vi "报警信息.vi"(8 "error in (no error)":errorcluster, 11 "data":T1) -> (0 "error out":errorcluster)   [LabVIEW 2016, in "MB SLAVE.lvlib"]
uses:
  MB SLAVE.lvlib
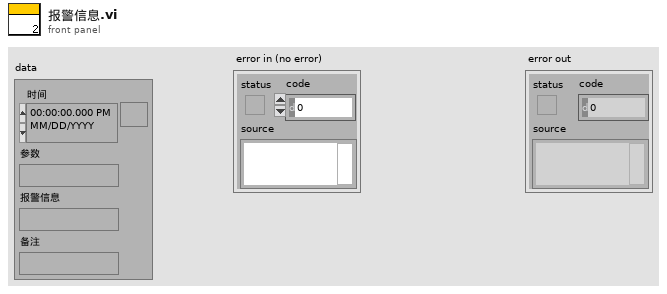
[diagram p1: front panel]
types:
  T1 = typedef "报警信息字段定义.ctl" = cluster{"时间":timestamp, "参数":string, "报警信息":string, "备注":string}
  T2 = typedef "数据库类型.ctl" = enum16{"Access", "SQLite"}
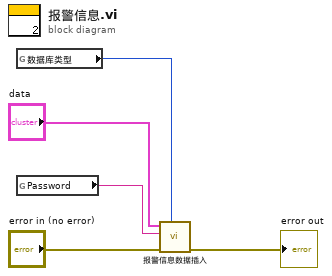
[diagram p0: block diagram]
diagram:
  n1 = global read "modbus slave全局.vi" "数据库类型"() -> (w3:T2)
  n2 = global read "modbus slave全局.vi" "Password"() -> (w1:string)
  n3 = call "报警信息数据插入.vi"("data"="data", "Password"=w1, "错误输入（无错误）"="error in (no error)", "数据库类型"=w3) -> ("错误输出"=→"error out":errorcluster)  [unwired: 6 in]
